vi "SaveOffsetGainVals.vi"(8 "error in":errorcluster, 11 "OffsetGain Array":dbl[](array[numeric])) -> (0 "error out":errorcluster)   [LabVIEW 2023, in "QSM - IODocs.lvlib"]
uses:
  QSM - IODocs.lvlib
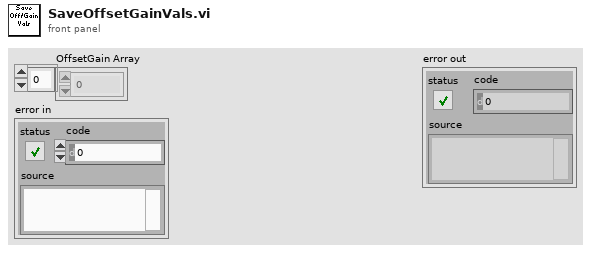
[diagram p1: front panel]
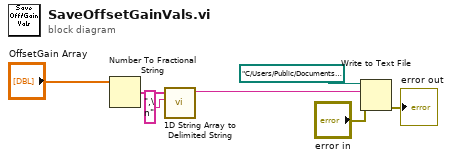
[diagram p0: block diagram]
diagram:
  n1 = Number To Fractional String(number="OffsetGain Array") -> (F-format string=w5:string[])  [unwired: 3 in]
  n2 = call <vilib>:"1D String Array to Delimited String.vi"("delimiter"=",\n", "string array"=w5) -> ("delimited string"=w3:string)  [unwired: 9 in]
  n3 = Write to Text File(file (use dialog)=path "C:/Users/Public/Documents/Grid2093/IO/OffsetGain.txt", text=w3, error in="error in") -> (error out=→"error out":errorcluster)  [unwired: 1 in, 2 out]
